vi "Spartan HTTP Run VI CGI.vi"(8 "error in (no error)":errorcluster, 9 "cgi/vit path":path, 10 "HTTP Data":T1 {"object data"."time" format="%0.2f"}) -> (0 "error out":errorcluster)   [LabVIEW 2011]
uses:
  Spartan HTTP Session.ctl
  Addons/internet/http/http_obj.llb/HTTP Session Data.ctl
  Addons/internet/utils/keyedarr.llb/Keyed Array.ctl
  server lib/Spartan CONFIG Global.vi
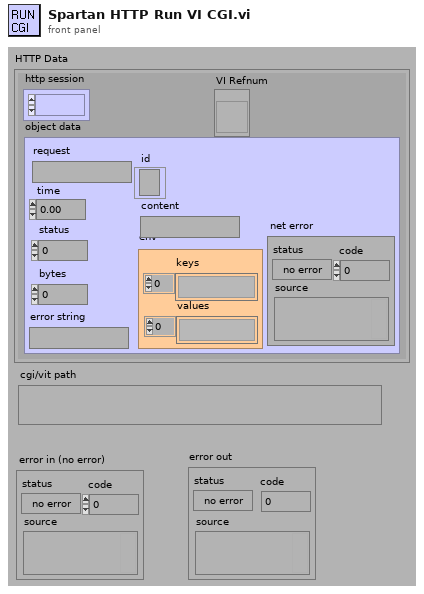
[diagram p1: front panel]
types:
  T1 = typedef "Spartan HTTP Session.ctl" = cluster{"http session":refnum<k1>, "object data":T2, "VI Refnum":refnum<vi>}
  T2 = typedef "HTTP Session Data.ctl" = cluster{"request":string, "time":dbl, "status":i32, "error string":string, "bytes":i32, "env":T3, "content":string, "id":refnum<k5>, "net error":errorcluster}
  T3 = typedef "Keyed Array.ctl" = cluster{"keys":string[], "values":string[]}
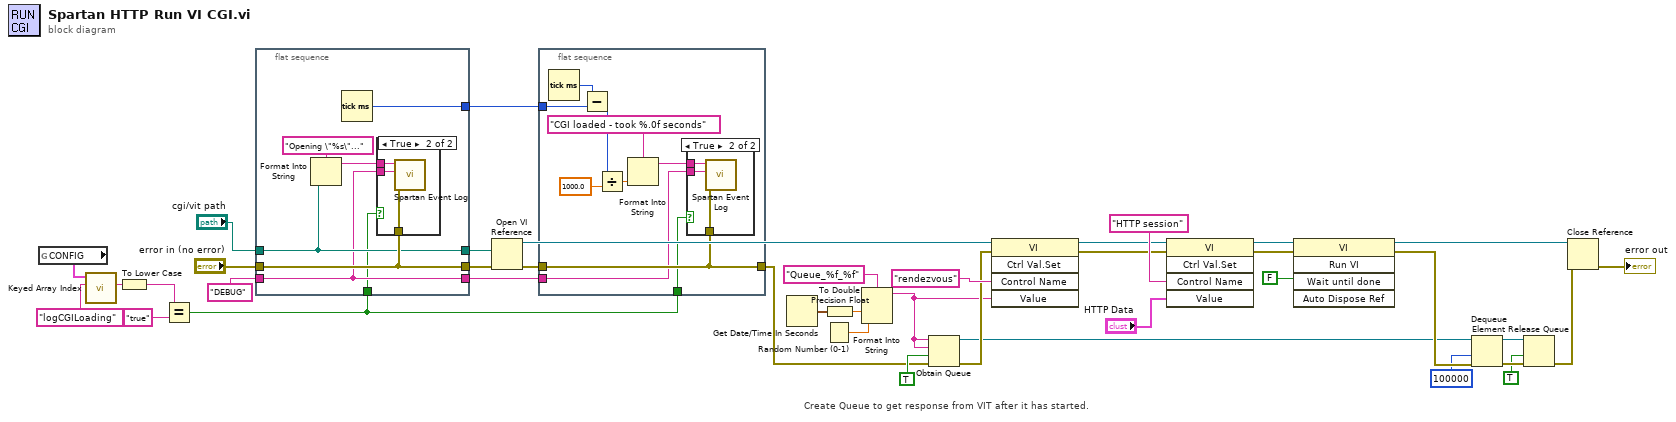
[diagram p0: block diagram]
diagram:
  # "Create Queue to get response from VIT after it has started."
  n1 = global read "Spartan CONFIG Global.vi" "CONFIG"() -> (w13:T3)
  n2 = call "Keyed Array Index.vi"("key"="logCGILoading" ("Control Name"), "array in"=w13) -> ("value"=w11:string)  [unwired: 2 in, 3 out]
  n3 = To Lower Case(string=w11) -> (all lower case string=w10:string)
  n4 = Equal?(x=w10, y="true") -> (x = y?=w1:bool)
  n5 = flat-sequence {
    tunnel: "error in (no error)" -> [w45]
    tunnel: "cgi/vit path" -> [w44]
    tunnel: [w45] -> w8
    tunnel: [w44] -> w7
    tunnel: "DEBUG" -> [w42]
    tunnel: [w43] -> w3
    tunnel: [w42] -> w2
    tunnel: w1 -> [w41]
    frame #0 {
      n6 = Format Into String(format string="Opening \"%s\"...", w44) -> (resulting string=w46:string)  [unwired: 2 in, 1 out]
      n7 = Tick Count (ms)() -> (millisecond timer value=w43:u32)
      n8 = case shown="True" w41 {
        tunnel: w46 -> [_ w50]
        tunnel: w45 -> [_ w49]
        tunnel: w42 -> [_ w48]
        frame False {
        }
        frame True {
          n9 = call "Spartan Event Log.vi"("error in (no error)"=w49, "module (\"\")"=w48, "message (\"\")"=w50) -> ()  [unwired: 5 in, 1 out]
        }
      }
    }
  }
  n10 = Open VI Reference(vi path=w7, error in (no error)=w8) -> (vi reference=w31:refnum<vi>, error out=w6:errorcluster)  [unwired: 2 in, 2 out]
  n11 = flat-sequence {
    tunnel: w6 -> [w58]
    tunnel: [w58] -> w5
    tunnel: w3 -> [w56]
    tunnel: w2 -> [w52]
    tunnel: w1 -> [w51]
    frame #0 {
      n12 = Tick Count (ms)() -> (millisecond timer value=w57:u32)
      n13 = Subtract(x=w57, y=w56) -> (x-y=w55:u32)
      n14 = Divide(x=w55, y=1000.0 ("x/y")) -> (x/y=w54:dbl)
      n15 = Format Into String(format string="CGI loaded - took %.0f seconds", w54) -> (resulting string=w59:string)  [unwired: 2 in, 1 out]
      n16 = case shown="True" w51 {
        tunnel: w59 -> [_ w63]
        tunnel: w58 -> [_ w62]
        tunnel: w52 -> [_ w61]
        frame False {
        }
        frame True {
          n17 = call "Spartan Event Log.vi"("error in (no error)"=w62, "module (\"\")"=w61, "message (\"\")"=w63) -> ()  [unwired: 5 in, 1 out]
        }
      }
    }
  }
  n18 = Get Date/Time In Seconds() -> (seconds since 1Jan1904=w27:timestamp)
  n19 = Random Number (0-1)() -> (number: 0 to 1=w25:dbl)
  n20 = To Double Precision Float(number=w27) -> (double precision float=w26:dbl)
  n21 = Format Into String(format string="Queue_%f_%f" ("Control Name"), w26, w25) -> (resulting string=w16:string)  [unwired: 2 in, 1 out]
  n22 = Obtain Queue(name (unnamed)=w16, element data type=w16, create if not found? (T)=TRUE ("return existing (F)"), error in (no error)=w5) -> (queue out=w19:refnum<queue>, error out=w20:errorcluster)  [unwired: 1 in, 1 out]
  n23 = invoke class="VI" method="Ctrl Val.Set"(reference=w31, error in=w20, "Control Name"="rendezvous", "Value"=w16) -> (reference out=w32:refnum<vi>, error out=w29:errorcluster)  [unwired: 1 in, 3 out]
  n24 = invoke class="VI" method="Ctrl Val.Set"(reference=w32, error in=w29, "Control Name"="HTTP session", "Value"="HTTP Data") -> (reference out=w36:refnum<vi>, error out=w38:errorcluster)  [unwired: 1 in, 3 out]
  n25 = invoke class="VI" method="Run VI"(reference=w36, error in=w38, "Wait until done"=FALSE) -> (reference out=w35:refnum<vi>, error out=w30:errorcluster)  [unwired: 2 in, 3 out]
  n26 = Dequeue Element(queue=w19, timeout in ms (-1)=100000 ("ms timeout (-1)"), error in (no error)=w30) -> (queue out=w18:refnum<queue>, error out=w22:errorcluster)  [unwired: 2 out]
  n27 = Release Queue(queue=w18, force destroy? (F)=TRUE ("return existing (F)"), error in (no error)=w22) -> (error out=w28:errorcluster)  [unwired: 2 out]
  n28 = Close Reference(reference=w35, error in (no error)=w28) -> (error out=→"error out":errorcluster)
